vi "603xA 662xA Read OVP Setting.vi"(8 "error in (no error)":errorcluster, 9 "channel (1)":u8=1 min=1 max=4 step=1, 11 "VISA resource name":refnum<visa-resource-name>) -> (0 "error out":errorcluster, 1 "OVP trip voltage":dbl format="%.4f", 3 "VISA resource name out":refnum<visa-resource-name>)   [LabVIEW 2020, in "Agilent 6XXX Series.lvlib"]
doc: "This function measures the Overvoltage Protection trip voltage."
uses:
  <instrlib>/Agilent 6XXX Series/Agilent 6XXX Series.lvlib
panel:
  # "HP603XA and HP662XA series only"
  # "*662xA only"
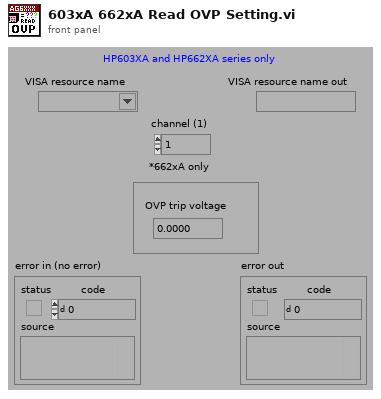
[diagram p1: front panel]
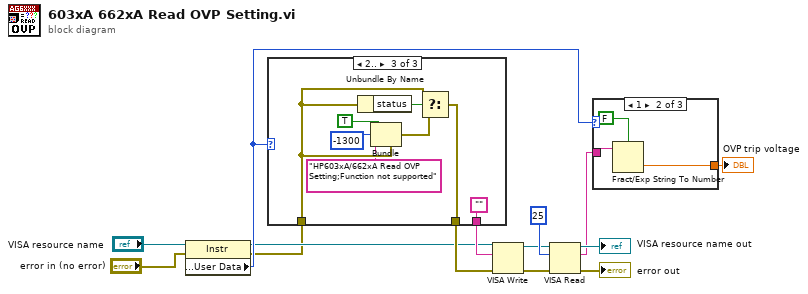
[diagram p0: block diagram]
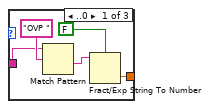
[diagram p2: hidden frame]
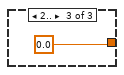
[diagram p3: hidden frame]
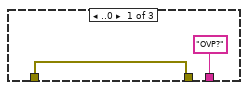
[diagram p4: hidden frame]
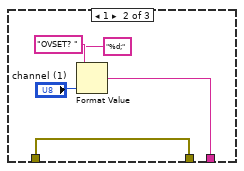
[diagram p5: hidden frame]
diagram:
  n1 = property class="Instr"(reference="VISA resource name", error in="error in (no error)") -> (reference out=w4:refnum<visa-resource-name>, error out=w3:errorcluster, "General Settings:User Data"=w7:u32)
  n2 = case shown="2.." w7 {
    tunnel: ["OVP?" w18 ""] -> w11
    tunnel: w3 -> [w15 w21 w26]
    tunnel: [w15 w21 w24] -> w10
    frame ..0 {
    }
    frame 1 {
      n3 = Format Value(string ("")="OVSET? ", format string="%d;", value (0)="channel (1)") -> (output string=w18:string)
    }
    frame 2.. {
      n4 = Unbundle By Name(w26) -> ("status"=w29:bool)
      n5 = Bundle(cluster=w26, "status"=TRUE, "code"=-1300, "source"="HP603xA/662xA Read OVP Setting;Function not supported") -> (w25:errorcluster)
      n6 = Select(t=w26, s=w29, f=w25) -> (s? t:f=w24:errorcluster)
    }
  }
  n7 = VISA Write(VISA resource name=w4, write buffer=w11, error in (no error)=w10) -> (VISA resource name out=w1:refnum<visa-resource-name>, error out=w2:errorcluster)  [unwired: 1 out]
  n8 = VISA Read(VISA resource name=w1, byte count=u32 25, error in (no error)=w2) -> (VISA resource name out=→"VISA resource name out":refnum<visa-resource-name>, read buffer=w9:string, error out=→"error out":errorcluster)  [unwired: 1 out]
  n9 = case shown="1" w7 {
    tunnel: w9 -> [w32 w36 _]
    tunnel: [w31 w37 0.0] -> w8
    frame ..0 {
      n10 = Match Pattern(string=w32, regular expression="OVP ") -> (after substring=w33:string)  [unwired: 1 in, 3 out]
      n11 = Fract/Exp String To Number(use system decimal point (T)=FALSE, string=w33) -> (number=w31:dbl)  [unwired: 2 in, 1 out]
    }
    frame 1 {
      n12 = Fract/Exp String To Number(use system decimal point (T)=FALSE, string=w36) -> (number=w37:dbl)  [unwired: 2 in, 1 out]
    }
    frame 2.. {
    }
  }
  "OVP trip voltage" <- w8
